vi "heron.vi"(9 "c":dbl=5.0, 10 "b":dbl=4.0, 11 "a":dbl=3.0) -> (3 "area":dbl)   [LabVIEW 2024]
doc: "Calculatess the area of triangle"
panel:
  out "output variable":dbl
  # "a) declaration of in/out parameters"
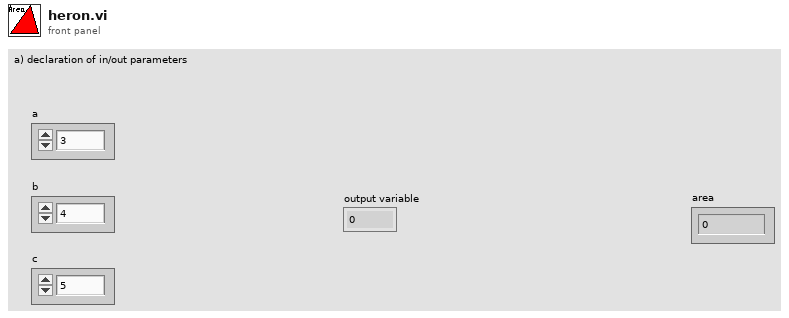
[diagram p1: front panel]
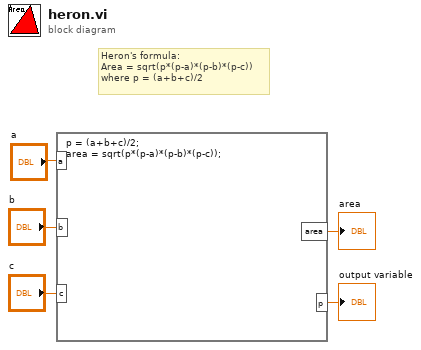
[diagram p0: block diagram]
diagram:
  # "Heron's formula:\nArea = sqrt(p*(p-a)*(p-b)*(p-c))\nwhere p = (a+b+c)/2"
  n1 = formula code="p = (a+b+c)/2;\narea = sqrt(p*(p-a)*(p-b)*(p-c));"("a"="a", "b"="b", "c"="c") -> ("area"=→"area":dbl, "p"=→"output variable":dbl)
